vi "CRYDecide InitIndex.vi"(10 "Steps In":T1[](array[typedef]) {"Repeat State Array"."Start" format="%#_5g"; "Y dB ref" format="%.1f"; "Y data" items=["dB", "Lin"]; "Start" format="%#_5g"}) -> ()   [LabVIEW 2013]
uses:
  Typedef Control/CRYStep.ctl
  Task Sequence/CRYProject Run Control Global.vi
  CRYStatistics Global.vi
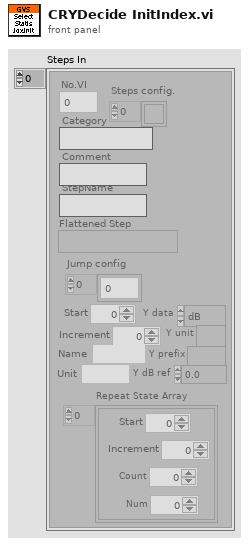
[diagram p1: front panel]
types:
  T1 = typedef "CRYStep.ctl" = cluster{"No.VI":i32, "Category":string, "StepName":string, "Seq setup flattened":string, "Comment":string, "Steps config.":bool[], "Jump config":i32[], "Start":dbl, "Increment":dbl, "Name":string, "Unit":string, "Y data":u16, "Y prefix":string, "Y dB ref":dbl, "Y unit":string, "Repeat State Array":cluster{"Start":dbl, "Increment":dbl, "Count":i32, "Num":i32}[]}
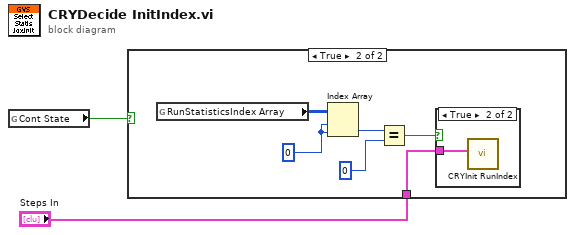
[diagram p0: block diagram]
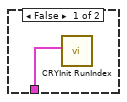
[diagram p2: hidden frame]
diagram:
  n1 = global read "CRYProject Run Control Global.vi" "Cont State"() -> (w2:bool)
  n2 = case shown="True" w2 {
    tunnel: "Steps In" -> [w3 w5]
    frame False {
      n3 = call "CRYInit RunIndex.vi"("Steps In"=w3) -> ()  [unwired: 11 in]
    }
    frame True {
      w4 = 0 ("index (row)")
      n4 = global read "CRYStatistics Global.vi" "RunStatisticsIndex Array"() -> (w9:u16[][])
      n5 = Index Array(array=w9, index (row)=w4, index (col)=w4) -> (element=w8:u16)
      n6 = Equal?(x=w8, y=u16 0) -> (x = y?=w6:bool)
      n7 = case shown="True" w6 {
        tunnel: w5 -> [_ w10]
        frame False {
        }
        frame True {
          n8 = call "CRYInit RunIndex.vi"("Steps In"=w10) -> ()  [unwired: 11 in]
        }
      }
    }
  }
